vi "Read MenuRef.vi"(8 "error in (no error)":errorcluster, 11 "Selector in":refnum<class "Selector.lvclass">) -> (0 "error out":errorcluster, 2 "MenuRef":refnum<k9>, 3 "Selector out":refnum<class "Selector.lvclass">)   [LabVIEW 2019, in "Selector.lvclass"]
uses:
  Selector.lvclass
  Selector.lvclass/Selector.ctl
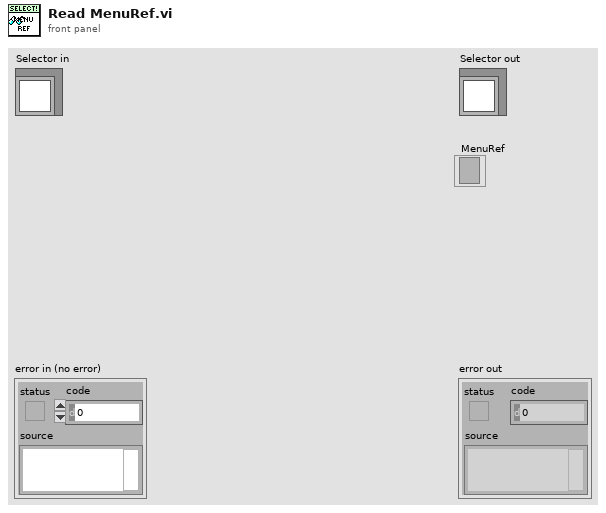
[diagram p1: front panel]
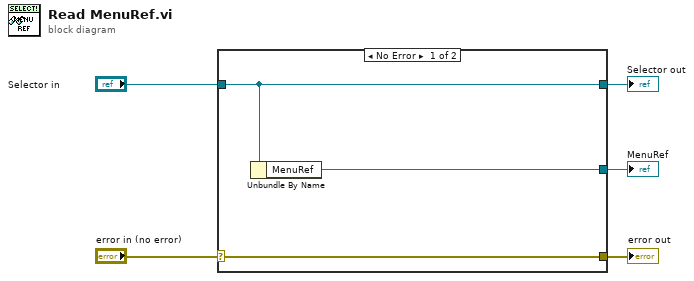
[diagram p0: block diagram]
diagram:
  n1 = case shown="No Error" "error in (no error)" {
    selector: "error in (no error)" -> [w8 w9]
    tunnel: [w8 w9] -> w4
    tunnel: [w7 w10] -> w2
    tunnel: "Selector in" -> [w7 w10]
    tunnel: [w6 _] -> w1
    frame No Error {
      n2 = Unbundle By Name(w7) -> ("MenuRef"=w6:refnum<k9>)
    }
    frame Error {
    }
  }
  "error out" <- w4
  "Selector out" <- w2
  "MenuRef" <- w1
